vi "Find Average Center.vi"(5 "Position":i32, 7 "Tray Number":i32, 8 "Assembly Type":string, 9 "XYZTheta":dbl[](array[numeric]), 11 "Gantry In":refnum<k24>) -> (1 "XYZTheta":dbl[](array[numeric]) format="%.6g", 3 "Gantry Out":refnum<k24>)   [LabVIEW 2021, in "Component Tray.lvclass"]
uses:
  Component Tray.lvclass
  Find Component.ctl
  Controller/Camera/Machine Vision.ctl
  C:/Program Files (x86)/Aerotech/A3200/LabVIEW/2010/Bin/Aerotech.A3200.dll
  Program Files (x86)/Aerotech/A3200/LabVIEW/2010/Bin/Aerotech.A3200.dll
  Controller/Camera/Image processing.ctl
  Controller/Camera/Camera settings.ctl
  Controller/Camera/Material.ctl
  Controller/Camera/Edmund Optics/Edmund Optics.lvclass
  C:/Users/User/Documents/Jessica_Code/Jessica_code_06052024/Gantry-CMU/UCSB-Gantry-HEP-main/Classes/Controller/Camera/Camera.lvclass
  Controller/Camera/Camera.lvclass
  Controller/Motion/A3200/A3200.lvclass
  Controller/Motion/Motion.lvclass
  Routine/TypeOfHexaboard.ctl
  Routine/Routine.lvclass
panel:
  out "Low Speed":bool
  out "X":bool
  out "Y":bool
  out "Z":bool
  out "High Speed":bool
  in  "Go to Top Right":bool
  in  "Go to Bottom Right":bool
  out "Program Stopped":bool
  out "XY Graph":cluster{"X":dbl, "Y":dbl}[](graph)
  out "Sensor ID Location":dbl[](array[numeric])
  in  "Go to Sensor ID":bool
  out "CH1 Location":dbl[](array[numeric])
  in  "Verify CH1":bool
  out "CH1 correct?":bool
  in  "Go to CH1":bool
  in  "Focus step size":dbl format="%#_13g"
  in  "number of focus steps":i32
  out "Average Strength":dbl
  in  "Focus":bool
  in  "Material":T1
  out "All fiducials recorded":bool
  in  "Override presets":bool
  in  "Camera settings":T2={"Gamma"=1.6, "Gain"=0, "Sharpness"=0, "Contrast"=0.0, "Exposure"=0.0078125} {"Exposure" min=0.000244140625 max=0.5 scale=0.0002..0.5; "Contrast" min=0.0 max=1.0 scale=0.001..1.0; "Sharpness" min=0 max=2 step=1 scale=0.0..2.0; "Gain" min=0 max=100 step=1 scale=0.1..100.0; "Gamma" min=0.01 max=10.0 scale=0.01..10.0}
  in  "Image processing":T3={"Brightness"=128.0, "Contrast"=45.0, "Gamma"=1.0471123} {"Brightness" scale=0.0..400.0; "Contrast" scale=0.0..90.0; "Gamma" scale=0.005..5.0}
  in  "Machine Vision":T4=enum."Sensor Fiducials"
  out "Gantry":dbl[](array[numeric]) format="%.6g"
  out "Sum":dbl[](array[numeric]) format="%.6g"
  out "Bottom Right XY":dbl[](array[numeric]) format="%.6g"
  out "Bottom Left XY":dbl[](array[numeric]) format="%.6g"
  out "Top Right XY":dbl[](array[numeric]) format="%.6g"
  out "Top Left XY":dbl[](array[numeric]) format="%.6g"
  in  "Record Bottom Left":bool
  in  "Record Bottom Right":bool
  in  "Record Top Right":bool
  in  "Record Top Left":bool
  in  "Go to Bottom Left":bool
  in  "Go to Top Left":bool
  in  "Joystick":bool
  out "Camera":dbl[](array[numeric]) format="%.6g"
  in  "Go to Center":bool
  in  "Component":T5
  in  "Stop Program":bool
  out "Image":T6(plugin-control)
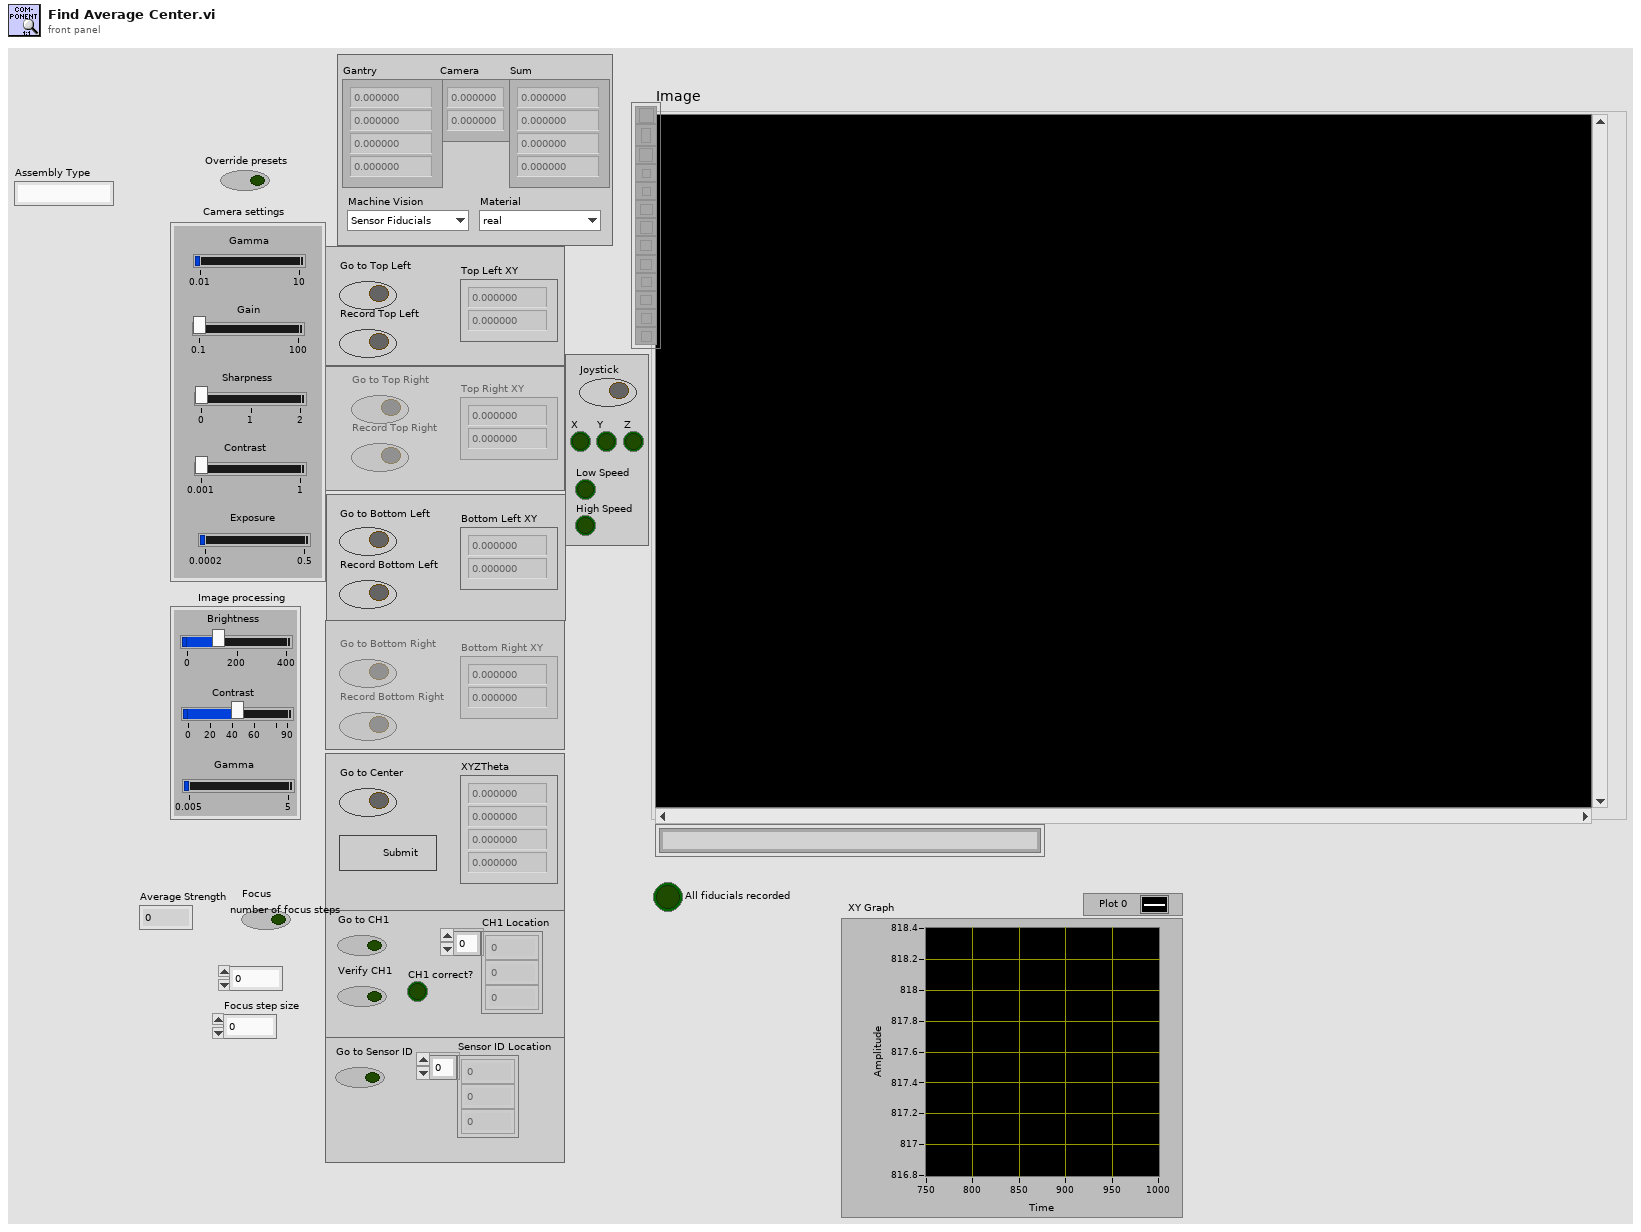
[diagram p1: front panel]
types:
  T1 = typedef "Camera.lvclass/Material.ctl" = enum16{"real", "dummy", "PETG"}
  T2 = typedef "Camera.lvclass/Camera settings.ctl" = cluster{"Gamma":dbl, "Gain":i64, "Sharpness":i64, "Contrast":dbl, "Exposure":dbl}
  T3 = typedef "Camera.lvclass/Image processing.ctl" = cluster{"Brightness":sgl, "Contrast":sgl, "Gamma":sgl}
  T4 = typedef "Camera.lvclass/Machine Vision.ctl" = enum16{"None", "Tray Fiducials", "Sensor Fiducials", "HPK Silicon", "Partial Hexaboard", "Partial Hexaboard Test", "100um dot", "Hexaboard", "Corner (TL, BR)", "Corner (BL, TR)", "V3 Sensor Cross", "V3 Sensor Circle", "test"}
  T5 = typedef "Component Tray.lvclass/Find Component.ctl" = cluster{"New Fiducials":dbl[], "Past Fiducials":dbl[], "XYZTheta":dbl[], "Fiducials Path":path, "Position":i32, "CH1 Location":dbl[], "Sensor ID Location":dbl[]}
  T6 = typedef "IMAQ Image.ctl" = refnum<image>
  T7 = typedef "Routine.lvclass/TypeOfHexaboard.ctl" = enum16{"Full Sensor", "Full PCB", "Right Partial PCB", "Right Partial Sensor", "Al Dummy Right Partial Sensor"}
  T8 = typedef "File Paths.ctl" = cluster{"Glue Pattern Folder":path, "Carrier Tray Folder":path, "Pick Up Tool Fixture Folder":path, "Components Folder":path, "Bellows Tool Offset.txt":path, "Pick Up Tool Offset.txt":path, "Dispense Tip Offset.txt":path, "Log Files":path, "Gantry Assembly Map.txt":path, "Syringe and offset map.txt":path, "Controllers Folder":path, "Local dbase config":path}
  T9 = enum8{"Enabled", "Disabled", "Disabled and Grayed Out"}
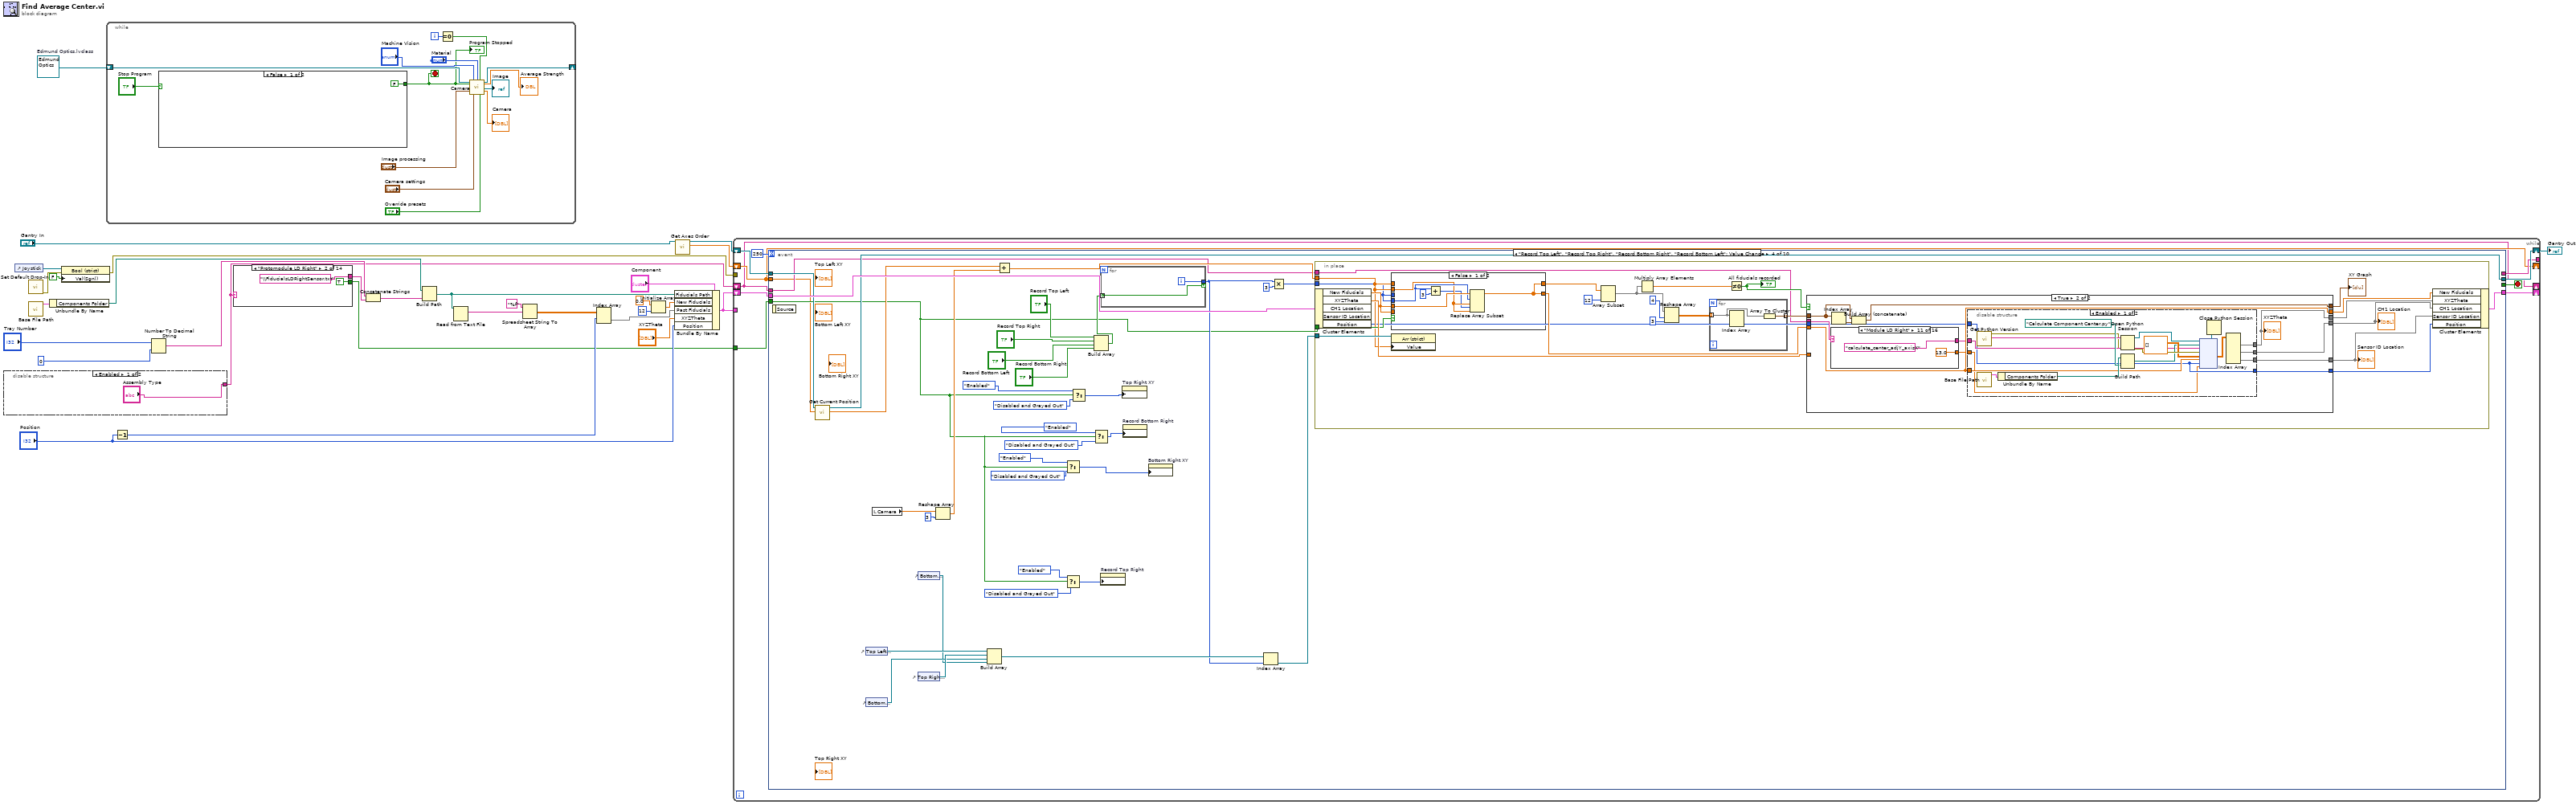
[diagram p0: block diagram]
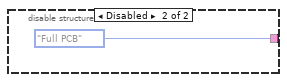
[diagram p2: hidden frame]
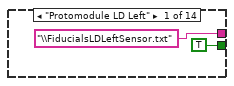
[diagram p3: hidden frame]
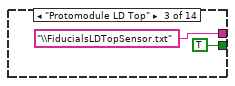
[diagram p4: hidden frame]
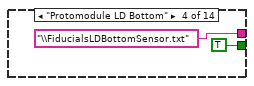
[diagram p5: hidden frame]
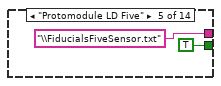
[diagram p6: hidden frame]
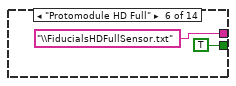
[diagram p7: hidden frame]
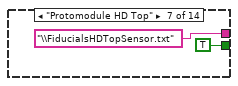
[diagram p8: hidden frame]
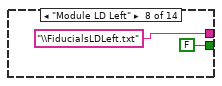
[diagram p9: hidden frame]
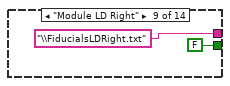
[diagram p10: hidden frame]
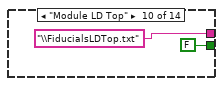
[diagram p11: hidden frame]
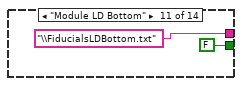
[diagram p12: hidden frame]
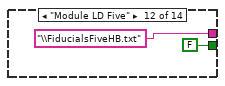
[diagram p13: hidden frame]
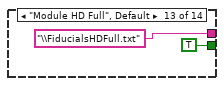
[diagram p14: hidden frame]
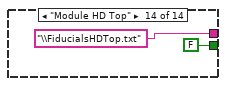
[diagram p15: hidden frame]
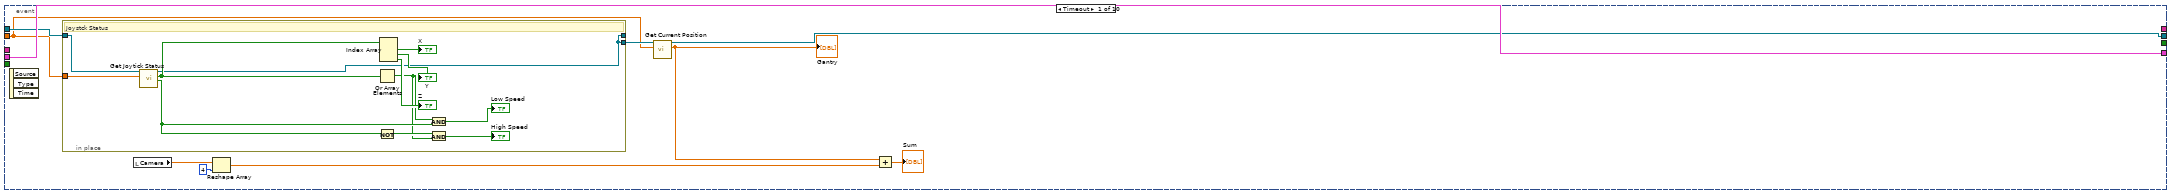
[diagram p16: hidden frame]
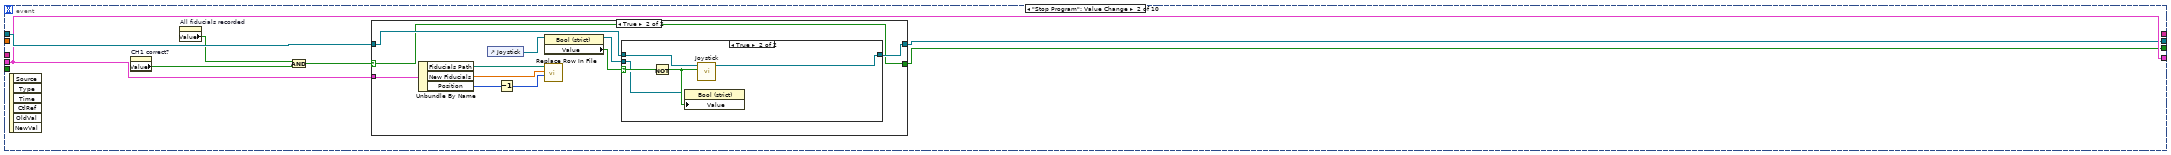
[diagram p17: hidden frame]
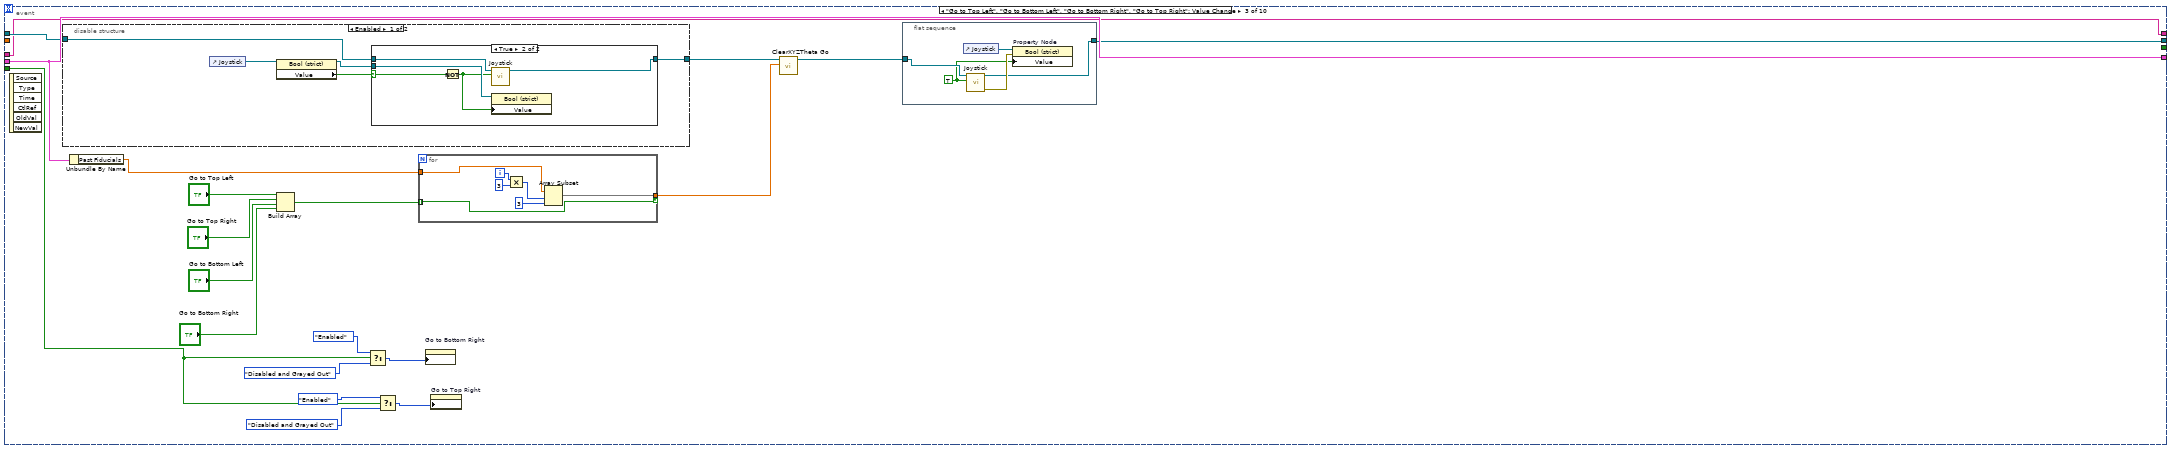
[diagram p20: hidden frame]
diagram:
  w27 = refnum<class "Edmund Optics.lvclass"> refnum  # Edmund Optics.lvclass
  n1 = disable-structure shown="Enabled" {
    disable-tunnel: ["Assembly Type" TypeOfHexaboard."Full PCB" ("Type of Hexaboard")] -> w5
    frame Enabled {
    }
    frame Disabled {
    }
  }
  n2 = control-ref of="Joystick"() -> (w30:refnum<vi>)
  n3 = call "Set Default Drop-In.vi"() -> ("error out"=w8:errorcluster)  [unwired: 11 in]
  n4 = call "Base File Path.vi"() -> ("Paths Out"=w18:T8)  [unwired: 11 in]
  n5 = Unbundle By Name(w18) -> ("Components Folder"=w20:path)
  n6 = property class="Bool (strict)"(reference=w30, error in=w8, "Val(Sgnl)"=FALSE) -> (error out=w28:errorcluster)  [unwired: 1 out]
  n7 = while {
    shift-right: [w43] -> _
    shift-left: w27 -> [w47]
    i -> [w39]
    stop <- w34 stop-if-true
    n8 = case shown="False" "Stop Program" {
      tunnel: [FALSE w49] -> w34
      frame False {
      }
      frame True {
        n9 = property on="All fiducials recorded" class="Bool (strict)"() -> ("Value"=w52:bool)  [unwired: 2 in, 2 out]
        n10 = property on="CH1 correct?" class="Bool (strict)"() -> ("Value"=w50:bool)  [unwired: 2 in, 2 out]
        n11 = And(x=w52, y=w50) -> (x .and. y?=w51:bool)
        n12 = case shown="False" w51 {
          tunnel: [FALSE TRUE] -> w49
          frame False {
            n13 = One Button Dialog(message="At least one fiducial not recorded or component orientation not verified.") -> ()  [unwired: 1 in, 1 out]
          }
          frame True {
            n14 = property on="All fiducials recorded" class="Bool (strict)"("Val(Sgnl)"=FALSE) -> ()  [unwired: 2 in, 2 out]
          }
        }
      }
    }
    "Program Stopped" <- w34
    n15 = Equal To 0?(x=w39) -> (x = 0?=w38:bool)
    n16 = call "Camera.vi"("Camera in"=w47, "Stop"=w34, "BCG Image Processing"="Image processing", "Machine Vision"="Machine Vision", "Camera settings"="Camera settings", "Material"="Material", "Loop 0"=w38, "Override presets"="Override presets") -> ("Camera out"=w43:refnum<class "Edmund Optics.lvclass">, "Average Strength"=→"Average Strength":dbl, "Image"=→"Image":T6, "Camera"=→"Camera":dbl[])  [unwired: 5 in, 3 out]
  }
  n17 = Decrement(x="Position") -> (x-1=w9:i32)
  n18 = Number To Decimal String(number="Tray Number", width (-)=i16 0) -> (decimal integer string=w21:string)
  n19 = case shown="\"Protomodule LD Right\"" w5 {
    tunnel: ["\\FiducialsLDLeftSensor.txt" ("string") "\\FiducialsLDRightSensor.txt" ("string") "\\FiducialsLDTopSensor.txt" ("string") "\\FiducialsLDBottomSensor.txt" ("string") "\\FiducialsFiveSensor.txt" ("string") "\\FiducialsHDFullSensor.txt" ("string") "\\FiducialsHDTopSensor.txt" ("string") "\\FiducialsLDLeft.txt" ("string") "\\FiducialsLDRight.txt" ("string") "\\FiducialsLDTop.txt" ("string") "\\FiducialsLDBottom.txt" ("string") "\\FiducialsFiveHB.txt" ("string") "\\FiducialsHDFull.txt" ("string") "\\FiducialsHDTop.txt" ("string")] -> w22
    tunnel: [TRUE TRUE TRUE TRUE TRUE TRUE TRUE FALSE FALSE FALSE FALSE FALSE TRUE FALSE] -> w4
    frame "Protomodule LD Left" {
    }
    frame "Protomodule LD Right" {
    }
    frame "Protomodule LD Top" {
    }
    frame "Protomodule LD Bottom" {
    }
    frame "Protomodule LD Five" {
    }
    frame "Protomodule HD Full" {
    }
    frame "Protomodule HD Top" {
    }
    frame "Module LD Left" {
    }
    frame "Module LD Right" {
    }
    frame "Module LD Top" {
    }
    frame "Module LD Bottom" {
    }
    frame "Module LD Five" {
    }
    frame "Module HD Full", Default {
    }
    frame "Module HD Top" {
    }
  }
  n20 = Concatenate Strings "Concatenate Strings"(w21, w22) -> (w23:string)
  n21 = Build Path(base path=w20, name or relative path=w23) -> (appended path=w12:path)
  n22 = Read from Text File(file (use dialog)=w12) -> (text=w24:string)  [unwired: 3 in, 3 out]
  n23 = Spreadsheet String To Array(format string="%f", spreadsheet string=w24) -> (array=w26:dbl[][])  [unwired: 2 in]
  n24 = Index Array "Index Array"(array=w26, index (row)=w9) -> (element=w16:dbl[])  [unwired: 1 in]
  n25 = Initialize Array(0.0 ("element"), 12 ("dimension size")) -> (w15:dbl[])
  n26 = Bundle By Name "Bundle By Name"(cluster="Component", "Fiducials Path"=w12, "New Fiducials"=w15, "Past Fiducials"=w16, "XYZTheta"="XYZTheta", "Position"="Position") -> (w6:T5)
  n27 = call "Get Axes Order.vi"("Gantry In"="Gantry In") -> ("Axes Order"=w1:dbl[], "Gantry Out"=w2:refnum<k24>)  [unwired: 8 in, 1 out]
  n28 = while {
    shift-right: [w92] -> _
    shift-left: w6 -> [w93]
    tunnel: w28 -> [_]
    shift-right: [w89] -> w7
    shift-left: w2 -> [w90]
    tunnel: w6 -> [_]
    tunnel: [w88] -> _
    tunnel: w4 -> [w87]
    shift-right: [w86] -> _
    shift-left: w1 -> [w86]
    shift-right: [w85] -> _
    shift-left: w5 -> [w85]
    stop <- w94 stop-if-true
    n29 = event shown="[3] \"Record Top Left\", \"Record Top Right\", \"Record Bottom Right\", \"Record Bottom Left\": Value Change" {
      selector: _ -> [_ _ _ _ _ _ _ _ _ _]
      dyn-events: _ -> [_ _ _ _ _ _ _ _ _ _]
      timeout: 250 -> [_ _ _ _ _ _ _ _ _ _]
      tunnel: [_ w120 _ _ _ _ _ _ _ _] -> w94
      tunnel: w93 -> [w103 w122 w159 w223 w344 w392 w399 w414 w429 w439]
      tunnel: [w103 w122 w159 w222 w344 w392 w399 w414 w429 w439] -> w92
      tunnel: w90 -> [w97 w123 w158 w214 w346 w391 w395 w410 w425 w440]
      tunnel: [w99 w121 w155 w212 w345 w389 w393 w408 w423 w440] -> w89
      tunnel: w85 -> [_ _ w152 w211 _ _ _ _ _ _]
      tunnel: [_ _ w152 _ _ _ _ _ _ _] -> w88
      tunnel: w87 -> [_ _ w143 w187 _ _ _ _ _ _]
      tunnel: w86 -> [w95 _ _ w186 w334 _ _ _ _ _]
      event Timeout {
        n30 = event-data() -> ()  [unwired: 1 in, 3 out]
        n31 = in-place {
          in-place-border: w97 -> [w116]
          in-place-border: [w105] -> _
          in-place-border: w95 -> [w115]
          in-place-border: [w105] -> w96
          # "Joystck Status"
          n32 = call "Get Joytick Status.vi"("Axes Order"=w115, "Gantry In"=w116) -> ("JoystickLowSpeedActive"=w109:bool, "Joystick Status"=w111:bool[], "Gantry Out"=w105:refnum<k24>)  [unwired: 6 in, 1 out]
          n33 = Or Array Elements(Boolean array=w111) -> (logical OR=w107:bool)
          n34 = Not(x=w109) -> (.not. x?=w108:bool)
          n35 = Index Array(array=w111) -> (element #1=→"X":bool, element #2=→"Y":bool, element #3=→"Z":bool)  [unwired: 3 in]
          n36 = And(x=w107, y=w109) -> (x .and. y?=→"Low Speed":bool)
          n37 = And(x=w108, y=w107) -> (x .and. y?=→"High Speed":bool)
        }
        n38 = local read "Camera"() -> (w102:dbl[])
        n39 = Reshape Array(w102, 4 ("dimension size")) -> (w100:dbl[])
        n40 = call "Get Current Position.vi"("Axes Order"=w95, "Gantry In"=w96) -> ("XYZTheta Out"=w98:dbl[], "Gantry Out"=w99:refnum<k24>)  [unwired: 7 in, 1 out]
        "Gantry" <- w98
        n41 = Add(x=w98, y=w100) -> (x+y=→"Sum":dbl[])
      }
      event "Stop Program": Value Change {
        n42 = event-data() -> ()  [unwired: 1 in, 6 out]
        n43 = property on="CH1 correct?" class="Bool (strict)"() -> ("Value"=w119:bool)  [unwired: 2 in, 2 out]
        n44 = property on="All fiducials recorded" class="Bool (strict)"() -> ("Value"=w118:bool)  [unwired: 2 in, 2 out]
        n45 = And(x=w118, y=w119) -> (x .and. y?=w117:bool)
        n46 = case shown="True" w117 {
          selector: w117 -> [w124 w133]
          tunnel: w123 -> [w125 w135]
          tunnel: w122 -> [_ w136]
          tunnel: [w125 w134] -> w121
          tunnel: [w124 w133] -> w120
          frame False {
          }
          frame True {
            n47 = Unbundle By Name(w136) -> ("Fiducials Path"=w130:path, "New Fiducials"=w129:dbl[], "Position"=w131:i32)
            n48 = control-ref of="Joystick"() -> (w127:refnum<vi>)
            n49 = Decrement(x=w131) -> (x-1=w132:i32)
            n50 = property class="Bool (strict)"(reference=w127) -> (reference out=w126:refnum<vi>, "Value"=w128:bool)  [unwired: 1 in, 1 out]
            n51 = call "Replace Row In File.vi"("Index"=w132, "Insert Array"=w129, "Path"=w130) -> ()  [unwired: 8 in, 1 out]
            n52 = case shown="True" w128 {
              selector: w128 -> [_ w142]
              tunnel: w135 -> [w137 w141]
              tunnel: [w137 w140] -> w134
              tunnel: w126 -> [_ w138]
              frame False {
              }
              frame True {
                n53 = Not(x=w142) -> (.not. x?=w139:bool)
                n54 = property class="Bool (strict)"(reference=w138, "Value"=w139) -> ()  [unwired: 1 in, 2 out]
                n55 = call "Joystick.vi"("Joystick"=w139, "Gantry In"=w141) -> ("Gantry Out"=w140:refnum<k24>)  [unwired: 8 in, 1 out]
              }
            }
          }
        }
      }
      event "Go to Top Left", "Go to Bottom Left", "Go to Bottom Right", "Go to Top Right": Value Change {
        n56 = event-data() -> ()  [unwired: 1 in, 6 out]
        n57 = disable-structure shown="Enabled" {
          disable-tunnel: w158 -> [w165 _]
          disable-tunnel: [w164 _] -> w157
          frame Enabled {
            n58 = control-ref of="Joystick"() -> (w163:refnum<vi>)
            n59 = property class="Bool (strict)"(reference=w163) -> (reference out=w166:refnum<vi>, "Value"=w167:bool)  [unwired: 1 in, 1 out]
            n60 = case shown="True" w167 {
              selector: w167 -> [_ w173]
              tunnel: w165 -> [w168 w171]
              tunnel: [w168 w169] -> w164
              tunnel: w166 -> [_ w172]
              frame False {
              }
              frame True {
                n61 = Not(x=w173) -> (.not. x?=w170:bool)
                n62 = call "Joystick.vi"("Joystick"=w170, "Gantry In"=w171) -> ("Gantry Out"=w169:refnum<k24>)  [unwired: 8 in, 1 out]
                n63 = property class="Bool (strict)"(reference=w172, "Value"=w170) -> ()  [unwired: 1 in, 2 out]
              }
            }
          }
          frame Disabled {
          }
        }
        n64 = Unbundle By Name(w159) -> ("Past Fiducials"=w161:dbl[])
        n65 = Build Array "Build Array"("Go to Top Left", "Go to Top Right", "Go to Bottom Left", "Go to Bottom Right") -> (w162:bool[])
        n66 = Select(t=T9."Enabled" ("Disabled"), s=w143, f=T9."Disabled and Grayed Out" ("Disabled")) -> (s? t:f=w144:T9)
        n67 = Select(t=T9."Enabled" ("Disabled"), s=w143, f=T9."Disabled and Grayed Out" ("Disabled")) -> (s? t:f=w147:T9)
        n68 = for {
          tunnel: w162 -> [w185] mode=indexing
          tunnel: w161 -> [w184]
          tunnel: [w179] -> w160 if=w185
          i -> [w182]
          n69 = Multiply(x=w182, y=3) -> (x*y=w180:i32)
          n70 = Array Subset "Array Subset"(array=w184, index=w180, length=3) -> (w179:dbl[])
        }
        n71 = property on="Go to Bottom Right" class="Bool"("DisabledEnum"=w144) -> ()  [unwired: 2 in, 2 out]
        n72 = property on="Go to Top Right" class="Bool"("DisabledEnum"=w147) -> ()  [unwired: 2 in, 2 out]
        n73 = call "ClearXYZTheta Go.vi"("XYZTheta In"=w160, "Gantry In"=w157) -> ("Gantry Out"=w156:refnum<k24>)  [unwired: 7 in, 2 out]
        n74 = flat-sequence {
          tunnel: w156 -> [w178]
          tunnel: [w175] -> w155
          frame #0 {
            w174 = TRUE
            n75 = control-ref of="Joystick"() -> (w177:refnum<vi>)
            n76 = call "Joystick.vi"("Joystick"=w174, "Gantry In"=w178) -> ("error out"=w176:errorcluster, "Gantry Out"=w175:refnum<k24>)  [unwired: 8 in]
            n77 = property on="Property Node" class="Bool (strict)"(reference=w177, error in=w176, "Value"=w174) -> ()  [unwired: 2 out]
          }
        }
      }
      event "Record Top Left", "Record Top Right", "Record Bottom Right", "Record Bottom Left": Value Change {
        n78 = event-data() -> ()  [unwired: 1 in, 1 out]
        n79 = call "Get Current Position.vi"("Axes Order"=w186, "Gantry In"=w214) -> ("XYZTheta Out"=w213:dbl[], "Gantry Out"=w212:refnum<k24>)  [unwired: 7 in, 1 out]
        n80 = control-ref of="Top Left XY"() -> (w209:refnum<vi>)
        n81 = control-ref of="Bottom Left XY"() -> (w207:refnum<vi>)
        n82 = local read "Camera"() -> (w217:dbl[])
        n83 = control-ref of="Bottom Right XY"() -> (w206:refnum<vi>)
        n84 = control-ref of="Top Right XY"() -> (w208:refnum<vi>)
        n85 = Reshape Array(w217, 3 ("dimension size")) -> (w216:dbl[])
        n86 = Build Array "Build Array"(w209, w208, w207, w206) -> (w221:refnum<vi>[])
        n87 = Add(x=w213, y=w216) -> (x+y=w215:dbl[])
        n88 = Select(t=T9."Enabled" ("Disabled"), s=w187, f=T9."Disabled and Grayed Out" ("Disabled")) -> (s? t:f=w188:T9)
        n89 = Select(t=T9."Enabled" ("Disabled"), s=w187, f=T9."Disabled and Grayed Out") -> (s? t:f=w198:T9)
        n90 = Select(t=T9."Enabled" ("Disabled"), s=w187, f=T9."Disabled and Grayed Out" ("Disabled")) -> (s? t:f=w192:T9)
        n91 = Select(t=T9."Enabled" ("Disabled"), s=w187, f=T9."Disabled and Grayed Out") -> (s? t:f=w196:T9)
        n92 = Build Array "Build Array"("Record Top Left", "Record Top Right", "Record Bottom Left", "Record Bottom Right") -> (w210:bool[])
        n93 = for {
          tunnel: w210 -> [w224] mode=indexing
          tunnel: [w225] -> w201 if=w224
          i -> [w225]
        }
        n94 = property on="Record Top Right" class="Bool"("DisabledEnum"=w198) -> ()  [unwired: 2 in, 2 out]
        n95 = property on="Top Right XY" class="Arr (strict)"("DisabledEnum"=w192) -> ()  [unwired: 2 in, 2 out]
        n96 = property on="Record Bottom Right" class="Bool"("DisabledEnum"=w196) -> ()  [unwired: 2 in, 2 out]
        n97 = property on="Bottom Right XY" class="Arr (strict)"("DisabledEnum"=w188) -> ()  [unwired: 2 in, 2 out]
        n98 = Index Array "Index Array"(array=w221, index=w201) -> (element=w220:refnum<vi>)
        n99 = Multiply(x=w201, y=3) -> (x*y=w218:i32)
        n100 = in-place {
          in-place-border: w218 -> [w229]
          in-place-border: w220 -> [w247]
          in-place-border: w215 -> [w230]
          in-place-border: w211 -> [w234]
          in-place-border: w187 -> [w232]
          n101 = in-place-cluster #1(w223) -> ("New Fiducials"=w231:dbl[], "XYZTheta"=w246:dbl[], "Position"=w227:i32)  [unwired: 2 out]
          n102 = case shown="False" w232 {
            tunnel: w231 -> [w255 _]
            tunnel: w229 -> [w254 _]
            tunnel: w230 -> [w253 _]
            tunnel: [w250 w256] -> w233
            tunnel: w231 -> [_ w259]
            tunnel: w230 -> [_ w258]
            tunnel: w229 -> [_ w257]
            tunnel: [w250 w256] -> w228
            frame False {
              n103 = Add(x=w254, y=3) -> (x+y=w251:i32)
              n104 = Replace Array Subset "Replace Array Subset"(array=w255, new element #1=w253, index #1=w254, new element #2=w253, index #2=w251) -> (w250:dbl[])
            }
            frame True {
              n105 = Replace Array Subset "Replace Array Subset"(array=w259, new element=w258, index=w257) -> (w256:dbl[])
            }
          }
          n106 = property class="Arr (strict)"(reference=w247, "Value"=w230) -> ()  [unwired: 1 in, 2 out]
          n107 = Array Subset "Array Subset"(array=w228, length=12) -> (w241:dbl[])  [unwired: 1 in]
          n108 = Multiply Array Elements(1:w241) -> (0:w244:dbl)
          n109 = Reshape Array "Reshape Array"(w241, 4 ("dimension size"), 3 ("dimension size")) -> (w238:dbl[][])
          n110 = for {
            tunnel: w238 -> [w260] mode=indexing
            tunnel: [w261] -> w237 mode=indexing
            n111 = Index Array(array=w260) -> ()  [unwired: 2 in, 2 out]
            n112 = Array To Cluster(array=w260) -> (cluster=w261:cluster{"[0]":dbl, "[1]":dbl})
          }
          n113 = Not Equal To 0?(x=w244) -> (x != 0?=w235:bool)
          "All fiducials recorded" <- w235
          n114 = case shown="True" w235 {
            tunnel: [w265 w271] -> w249
            tunnel: w233 -> [w266 w275]
            tunnel: [w266 w275] -> w248
            tunnel: w246 -> [w265 _]
            tunnel: [w264 w272] -> w243
            tunnel: [w264 w273] -> w242
            tunnel: w237 -> [w263 w278]
            tunnel: [w263 w276] -> w236
            tunnel: w234 -> [_ w274]
            tunnel: w227 -> [w262 w269]
            tunnel: [w262 w268] -> w226
            frame False {
              w264 = dbl[] [] ("CH1 location")
            }
            frame True {
              n115 = case shown="\"Module LD Right\"" w274 {
                tunnel: ["calculate_center" ("function name") "calculate_center_adjY_axisY" ("function name") "calculate_center_adjY_axisY" ("function name") "calculate_center_adjX_axisY" ("function name") "calculate_center_adjX_axisY" ("function name") "calculate_center" ("function name") "calculate_center" ("function name") "calculate_center_adjX_axisY" ("function name") "calculate_center" ("function name") "calculate_center_adjY_axisX" ("function name") "calculate_center_adjY_axisX" ("function name") "calculate_center_adjX_axisY" ("function name") "calculate_center_adjX_axisY" ("function name") "calculate_center_adjY_axisX" ("function name") "calculate_center" ("function name") "calculate_center_adjX_axisY" ("function name")] -> w270
                tunnel: [0.0 -45.14 45.14 41.64 -41.64 0.0 0.0 49.78 0.0 -2.0 13.0 2.0 -1.38 0.0 0.0 21.0] -> w267
                frame "Protomodule LD Full", Default {
                }
                frame "Protomodule LD Left" {
                }
                frame "Protomodule LD Right" {
                }
                frame "Protomodule LD Top" {
                }
                frame "Protomodule LD Bottom" {
                }
                frame "Protomodule LD Five" {
                }
                frame "Protomodule HD Full" {
                }
                frame "Protomodule HD Top" {
                }
                frame "Module LD Full" {
                }
                frame "Module LD Left" {
                }
                frame "Module LD Right" {
                }
                frame "Module LD Top" {
                }
                frame "Module LD Bottom" {
                }
                frame "Module LD Five" {
                }
                frame "Module HD Full" {
                }
                frame "Module HD Top" {
                }
              }
              n116 = Index Array(array=w278) -> (element=w277:cluster{"[0]":dbl, "[1]":dbl})  [unwired: 1 in]
              n117 = Build Array (concatenate)(w278, w277) -> (w276:cluster{"[0]":dbl, "[1]":dbl}[])
              n118 = disable-structure shown="Enabled" {
                disable-tunnel: w275 -> [w288 w298]
                disable-tunnel: [w284 w301] -> w273
                disable-tunnel: [w285 w300] -> w272
                disable-tunnel: [w286 w299] -> w271
                disable-tunnel: w270 -> [w283 _]
                disable-tunnel: w269 -> [w280 _]
                disable-tunnel: [w280 _] -> w268
                disable-tunnel: w267 -> [w279 _]
                frame Enabled {
                  n119 = call "Get Python Version.vi"() -> ("Python Version"=w282:string, "error out"=w281:errorcluster)  [unwired: 10 in]
                  n120 = call "Base File Path.vi"() -> ("Paths Out"=w293:T8)  [unwired: 11 in]
                  n121 = Unbundle By Name(w293) -> ("Components Folder"=w291:path)
                  n122 = Open Python Session(python version=w282, 3:w281) -> (session out=w297:refnum<k35>, error out=w295:errorcluster)  [unwired: 1 in]
                  n123 = Build Path(base path=w291, name or relative path=path "Calculate Component Center.py") -> (appended path=w290:path)
                  n124 = node(w297, w290, w283, w295, dbl[][] [], w288, w280, w279) -> (w296:refnum<k35>, w294:errorcluster, w287:dbl[][])  [unwired: 3 in, 2 out]
                  n125 = Close Python Session(session in=w296, error in=w294) -> ()  [unwired: 1 out]
                  n126 = Index Array(array=w287) -> (element #1=w286:dbl[], element #2=w285:dbl[], element #3=w284:dbl[])  [unwired: 6 in]
                }
                frame Disabled {
                  n127 = call "Calculate Average Center.vi"("Gantry Fiducials"=w298) -> ("Sensor ID Location"=w301:dbl[], "CH1 Location"=w300:dbl[], "XYZTheta"=w299:dbl[])  [unwired: 8 in]
                }
              }
              "XYZTheta" <- w271
            }
          }
          "CH1 Location" <- w243
          "Sensor ID Location" <- w242
          "XY Graph" <- w236
          n128 = in-place-cluster #1("New Fiducials"=w248, "XYZTheta"=w249, "CH1 Location"=w243, "Sensor ID Location"=w242, "Position"=w226) -> (w222:T5)
        }
      }
      event "Focus": Value Change {
        n129 = event-data() -> ()  [unwired: 1 in, 6 out]
        n130 = Divide(x="number of focus steps", y=2) -> (x/y=w349:dbl)
        n131 = Multiply(x=w349, y="Focus step size") -> (x*y=w347:dbl)
        n132 = call "Joystick.vi"("Joystick"=FALSE, "Gantry In"=w346) -> ("Gantry Out"=w340:refnum<k24>)  [unwired: 8 in, 1 out]
        n133 = Negate(x=w347) -> (-x=w341:dbl)
        n134 = call "Z Go.vi"("Increment"=TRUE, "Return Immediately"=FALSE ("Increment"), "Speed In"=1.0 ("Speed"), "Position In"=w341, "Gantry In"=w340) -> ("error out"=w338:errorcluster, "Gantry Out"=w339:refnum<k24>)  [unwired: 3 in, 2 out]
        n135 = for {
          N: "number of focus steps" -> [_]
          tunnel: [w367] -> w360 mode=indexing
          tunnel: w338 -> [w366]
          tunnel: [w364] -> w353
          shift-right: [w368] -> w354
          shift-left: w339 -> [w370]
          tunnel: "Focus step size" -> [w363]
          tunnel: w334 -> [w362]
          n136 = flat-sequence {
            tunnel: w370 -> [w378]
            tunnel: [w377] -> w369
            tunnel: w366 -> [w376]
            tunnel: [w375] -> w365
            tunnel: w363 -> [w373]
            tunnel: w369 -> [w388]
            tunnel: [w387] -> w368
            tunnel: [w386] -> w367
            tunnel: w365 -> [w382]
            tunnel: [w381] -> w364
            tunnel: w362 -> [w379]
            frame #0 {
              n137 = call "Z Go.vi"("Increment"=TRUE, "Return Immediately"=FALSE ("Increment"), "error in (no error)"=w376, "Speed In"=0.1 ("Speed"), "Position In"=w373, "Gantry In"=w378) -> ("error out"=w375:errorcluster, "Gantry Out"=w377:refnum<k24>)  [unwired: 2 in, 2 out]
            }
            frame #1 {
              n138 = call "Get Current Position.vi"("error in (no error)"=w382, "Axes Order"=w379, "Gantry In"=w388) -> ("error out"=w381:errorcluster, "XYZTheta Out"=w385:dbl[], "Gantry Out"=w387:refnum<k24>)  [unwired: 6 in]
              n139 = local read "Average Strength"() -> (w380:dbl)
              n140 = Delete From Array(array=w385, index=2) -> (deleted portion=w383:dbl)  [unwired: 1 in, 1 out]
              n141 = Build Array(w380, w383) -> (w386:dbl[])
            }
          }
        }
        n142 = Transpose 2D Array(2D array=w360) -> (transposed array=w359:dbl[][])
        n143 = Index Array(array=w359) -> (element #2=w358:dbl[])  [unwired: 4 in, 1 out]
        n144 = Index Array(array=w359) -> (element=w361:dbl[])  [unwired: 2 in]
        n145 = Array Max & Min(array=w361) -> (max index (indices)=w357:i32)  [unwired: 3 out]
        n146 = Index Array(array=w358, index=w357) -> (element=w356:dbl)
        n147 = call "Z Go.vi"("Increment"=FALSE, "Return Immediately"=FALSE ("Increment"), "error in (no error)"=w353, "Speed In"=15.0 ("Speed"), "Position In"=w356, "Gantry In"=w354) -> ("Gantry Out"=w345:refnum<k24>)  [unwired: 2 in, 3 out]
      }
      event "Joystick": Value Change {
        n148 = event-data() -> ()  [unwired: 1 in, 6 out]
        n149 = call "Joystick.vi"("Joystick"="Joystick", "Gantry In"=w391) -> ("Gantry Out"=w389:refnum<k24>)  [unwired: 8 in, 1 out]
      }
      event "Go to Center": Value Change {
        n150 = event-data() -> ()  [unwired: 1 in, 6 out]
        n151 = Unbundle By Name(w399) -> ("XYZTheta"=w400:dbl[])
        n152 = control-ref of="Joystick"() -> (w396:refnum<vi>)
        n153 = property class="Bool (strict)"(reference=w396) -> (reference out=w397:refnum<vi>, "Value"=w398:bool)  [unwired: 1 in, 1 out]
        n154 = case shown="True" w398 {
          selector: w398 -> [_ w407]
          tunnel: w395 -> [w401 w404]
          tunnel: [w401 w403] -> w394
          tunnel: w397 -> [_ w406]
          frame False {
          }
          frame True {
            n155 = Not(x=w407) -> (.not. x?=w402:bool)
            n156 = call "Joystick.vi"("Joystick"=w402, "Gantry In"=w404) -> ("error out"=w405:errorcluster, "Gantry Out"=w403:refnum<k24>)  [unwired: 8 in]
            n157 = property class="Bool (strict)"(reference=w406, error in=w405, "Value"=w402) -> ()  [unwired: 2 out]
          }
        }
        n158 = call "ClearXYZTheta Go.vi"("XYZTheta In"=w400, "Gantry In"=w394) -> ("Gantry Out"=w393:refnum<k24>)  [unwired: 7 in, 2 out]
      }
      event "Go to CH1": Value Change {
        n159 = event-data() -> ()  [unwired: 1 in, 6 out]
        n160 = Unbundle By Name(w414) -> ("CH1 Location"=w415:dbl[])
        n161 = control-ref of="Joystick"() -> (w411:refnum<vi>)
        n162 = property class="Bool (strict)"(reference=w411) -> (reference out=w412:refnum<vi>, "Value"=w413:bool)  [unwired: 1 in, 1 out]
        n163 = case shown="True" w413 {
          selector: w413 -> [_ w422]
          tunnel: w410 -> [w416 w419]
          tunnel: [w416 w418] -> w409
          tunnel: w412 -> [_ w421]
          frame False {
          }
          frame True {
            n164 = Not(x=w422) -> (.not. x?=w417:bool)
            n165 = call "Joystick.vi"("Joystick"=w417, "Gantry In"=w419) -> ("error out"=w420:errorcluster, "Gantry Out"=w418:refnum<k24>)  [unwired: 8 in]
            n166 = property class="Bool (strict)"(reference=w421, error in=w420, "Value"=w417) -> ()  [unwired: 2 out]
          }
        }
        n167 = call "ClearXYZTheta Go.vi"("XYZTheta In"=w415, "Gantry In"=w409) -> ("Gantry Out"=w408:refnum<k24>)  [unwired: 7 in, 2 out]
      }
      event "Go to Sensor ID": Value Change {
        n168 = event-data() -> ()  [unwired: 1 in, 6 out]
        n169 = Unbundle By Name(w429) -> ("Sensor ID Location"=w430:dbl[])
        n170 = control-ref of="Joystick"() -> (w426:refnum<vi>)
        n171 = property class="Bool (strict)"(reference=w426) -> (reference out=w427:refnum<vi>, "Value"=w428:bool)  [unwired: 1 in, 1 out]
        n172 = case shown="True" w428 {
          selector: w428 -> [_ w437]
          tunnel: w425 -> [w431 w434]
          tunnel: [w431 w433] -> w424
          tunnel: w427 -> [_ w436]
          frame False {
          }
          frame True {
            n173 = Not(x=w437) -> (.not. x?=w432:bool)
            n174 = call "Joystick.vi"("Joystick"=w432, "Gantry In"=w434) -> ("error out"=w435:errorcluster, "Gantry Out"=w433:refnum<k24>)  [unwired: 8 in]
            n175 = property class="Bool (strict)"(reference=w436, error in=w435, "Value"=w432) -> ()  [unwired: 2 out]
          }
        }
        n176 = call "ClearXYZTheta Go.vi"("XYZTheta In"=w430, "Gantry In"=w424) -> ("Gantry Out"=w423:refnum<k24>)  [unwired: 7 in, 2 out]
      }
      event "Verify CH1": Value Change {
        n177 = event-data() -> ()  [unwired: 1 in, 6 out]
        "CH1 correct?" <- TRUE
      }
    }
  }
  "Gantry Out" <- w7
